vi "TCP Send Message.vi"(8 "error in":errorcluster, 9 "Timeout (ms)":i32=50, 10 "TCP-Message in":T1, 11 "Connection ID":refnum<k5>) -> (0 "error out":errorcluster, 2 "Bytes written":i32, 3 "Connection ID out":refnum<k5>)   [LabVIEW 2020, in "hse-network.lvlib"]
doc: "Send a message (measurement data, command, ...) via TCP. The message must be flattened to a string and the message typ is determined by the \"Message Type Enum\".\n\n____\nHAMPEL SOFTWARE ENGINEERING v3.8.0 (2023-12-18 14:41)"
uses:
  hse-network.lvlib
  TCP Message.ctl
  Message Types Enum.ctl
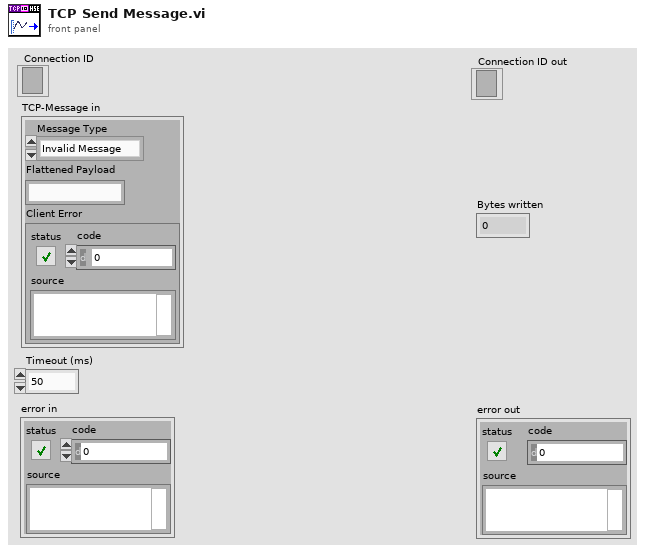
[diagram p1: front panel]
types:
  T1 = typedef "hse-network.lvlib/TCP Message.ctl" = cluster{"Message Type":T2, "Flattened Payload":string, "Client Error":errorcluster}
  T2 = typedef "hse-network.lvlib/Message Types Enum.ctl" = enum8{"Invalid Message", "Check-Message", "MHL-Command", "String", "1D-Array Wfm", "2D-Array DBL", "2D-Array I32"}
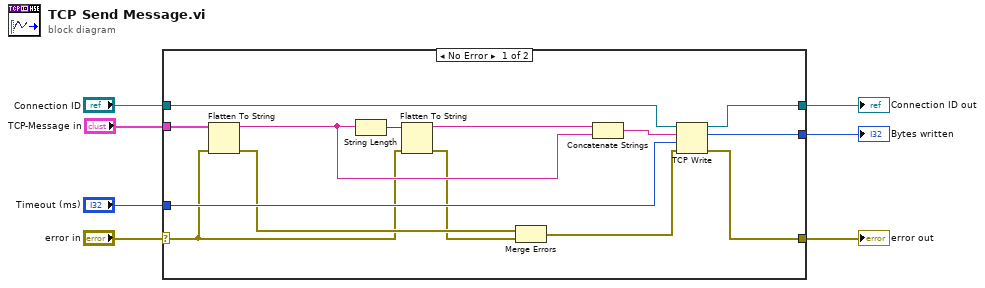
[diagram p0: block diagram]
diagram:
  n1 = case shown="No Error" "error in" {
    selector: "error in" -> [w10 w23]
    tunnel: [w21 w22] -> w7
    tunnel: "Connection ID" -> [w15 w22]
    tunnel: "Timeout (ms)" -> [w19 _]
    tunnel: [w8 w23] -> w3
    tunnel: [w18 _] -> w2
    tunnel: "TCP-Message in" -> [w14 _]
    frame No Error {
      n2 = Flatten To String(anything=w14, error in (no error)=w10) -> (data string=w13:string, error out=w12:errorcluster)  [unwired: 2 in, 1 out]
      n3 = String Length(string=w13) -> (length=w20:i32)
      n4 = Flatten To String(anything=w20, error in (no error)=w10) -> (data string=w17:string, error out=w11:errorcluster)  [unwired: 2 in, 1 out]
      n5 = Merge Errors(w12, w11) -> (w9:errorcluster)
      n6 = Concatenate Strings(w17, w13) -> (w16:string)
      n7 = TCP Write(connection ID=w15, data in=w16, error in (no error)=w9, 9:w19) -> (connection ID out=w21:refnum<k5>, bytes written=w18:i32, error out=w8:errorcluster)
    }
    frame Error {
    }
  }
  "error out" <- w3
  "Connection ID out" <- w7
  "Bytes written" <- w2
